vi "waveformprepare.vi"(7 "1762 Expose (us)":dbl, 8 "Microwave Expose Time (us)":dbl, 9 "Pump Expose Time (us)":dbl=256.0 format="%.2f") -> (3 "digital waveform out":digitalwaveform(waveform)={"t0"=timestamp(0 s since 1904-01-01), "dt"=0.0, "Y"={"transitions"=[], "data"=[]}, "error"={"status"=FALSE, "code"=37421928, "source"=""}})   [LabVIEW 2009]
uses:
  <vilib>/Waveform/DWDTOps.llb/DWDT Append Digital Samples.vi
  <vilib>/Waveform/DWDTOps.llb/DWDT Append Digital Signals.vi
  <vilib>/Waveform/DWDTOps.llb/Digital Pattern Generator (Single Value).vi
  <vilib>/Waveform/DWDTOps.llb/DWDT Invert Digital.vi
panel:
  out "Mixed Signal Graph":digitalwaveform(graph)
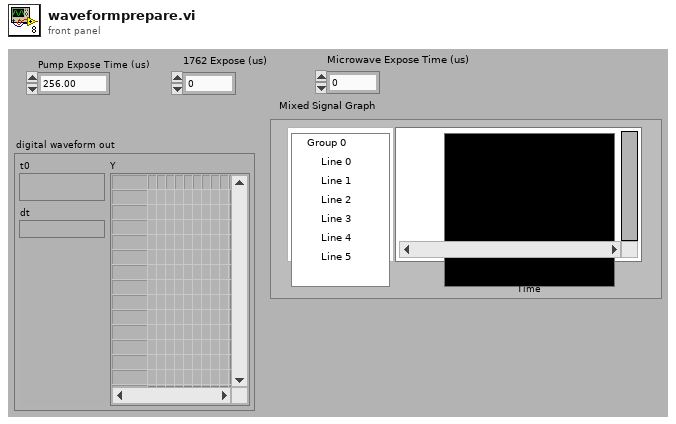
[diagram p1: front panel]
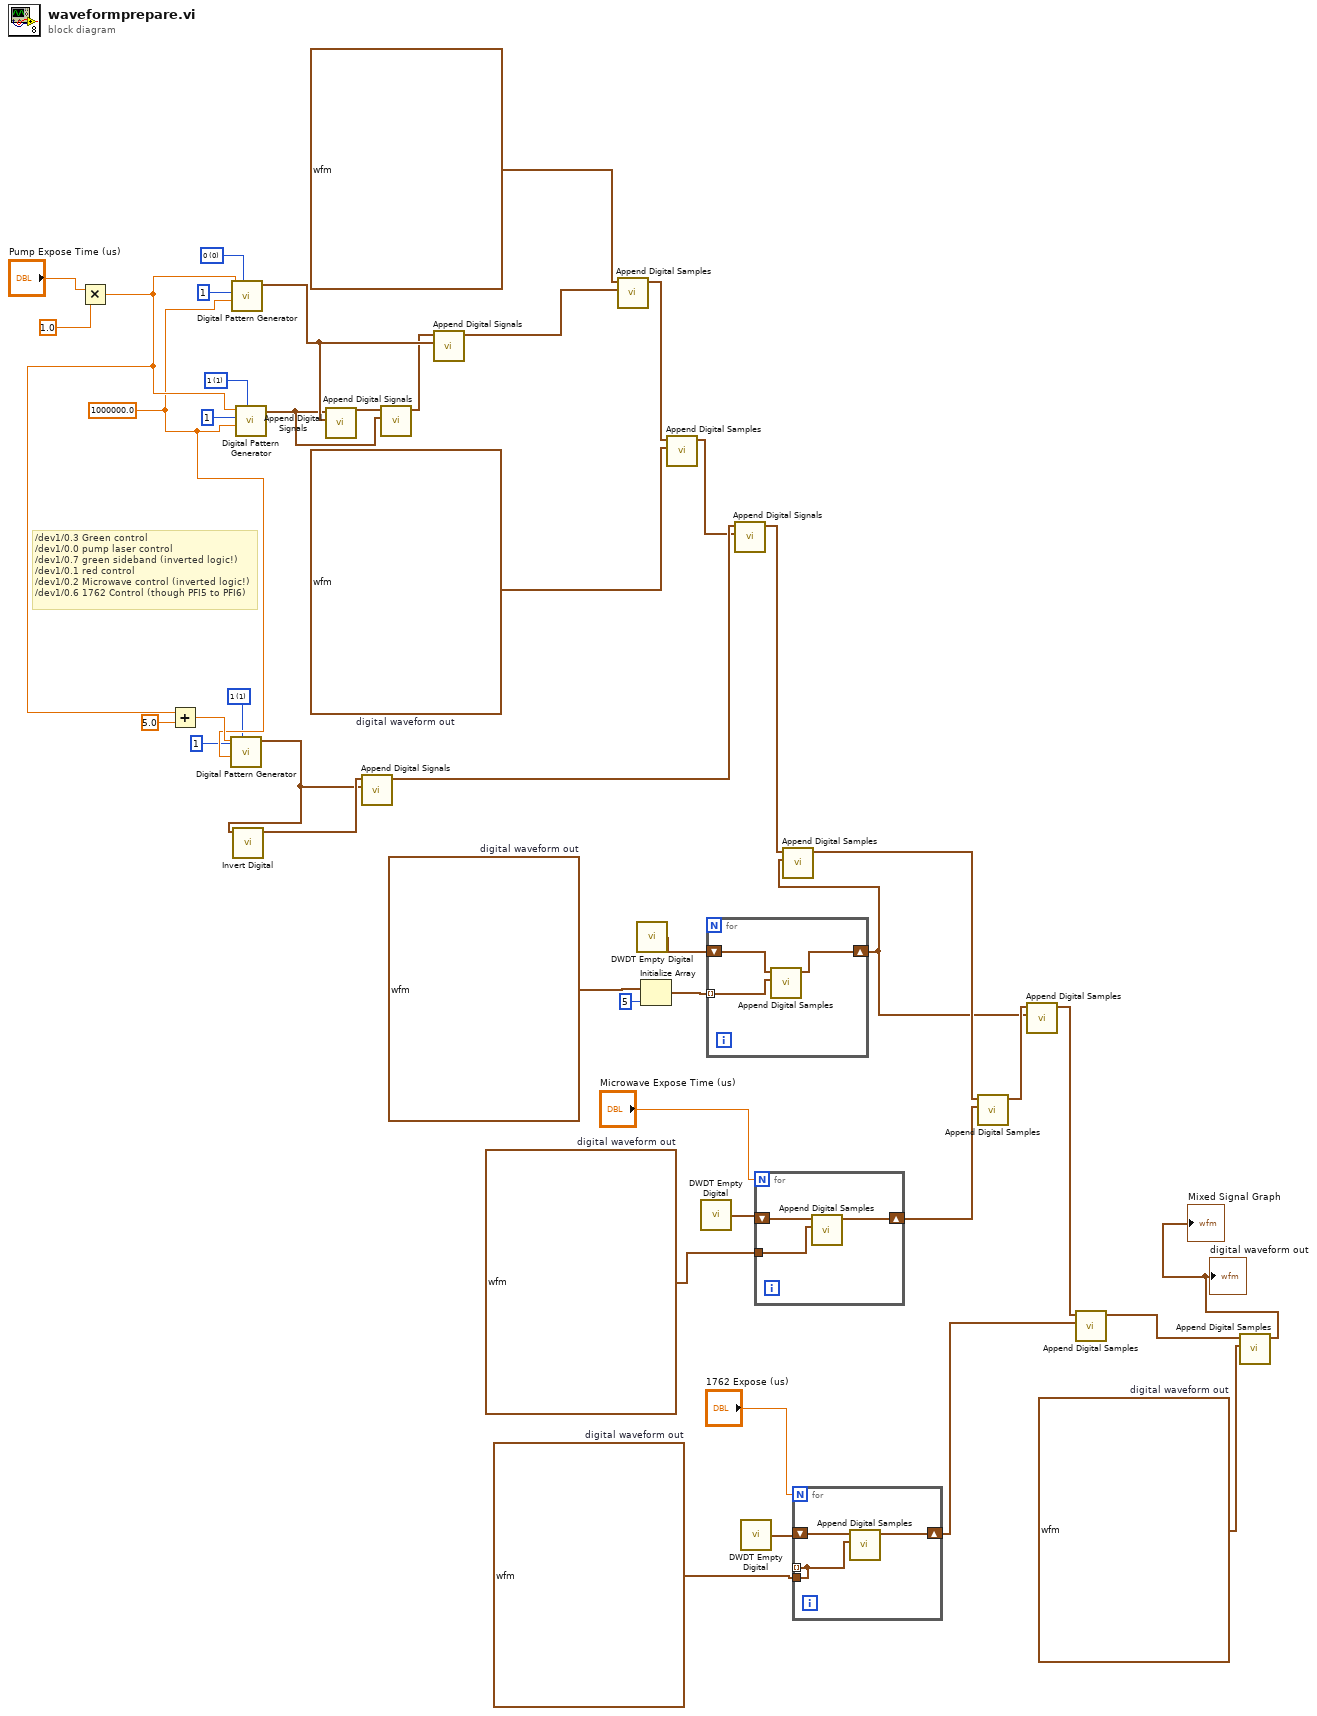
[diagram p0: block diagram]
diagram:
  w3 = digitalwaveform {"t0"=timestamp(0 s since 1904-01-01), "dt"=1e-06, "Y"={"transitions"=[], "data"=[[0, 1, 0, 1, 0, 0]]}, "error"={"status"=FALSE, "code"=37421928, "source"=""}}  # digital waveform out
  w11 = digitalwaveform {"t0"=timestamp(0 s since 1904-01-01), "dt"=1e-06, "Y"={"transitions"=[], "data"=[[1, 1, 0, 1, 0, 0]]}, "error"={"status"=FALSE, "code"=37421928, "source"=""}}  # digital waveform out
  w15 = digitalwaveform {"t0"=timestamp(0 s since 1904-01-01), "dt"=1e-06, "Y"={"transitions"=[], "data"=[[0, 0, 0, 1, 0, 0]]}, "error"={"status"=FALSE, "code"=37421928, "source"=""}}  # digital waveform out
  w19 = digitalwaveform {"t0"=timestamp(0 s since 1904-01-01), "dt"=1e-06, "Y"={"transitions"=[], "data"=[[0, 1, 0, 1, 0, 0]]}, "error"={"status"=FALSE, "code"=37421928, "source"=""}}  # digital waveform out
  w26 = u8 1 items=["0", "1", "Z", "L", "H", "X", "T", "V"] ("value")
  w39 = u8 1 items=["0", "1", "Z", "L", "H", "X", "T", "V"] ("value")
  w41 = u8 0 items=["0", "1", "Z", "L", "H", "X", "T", "V"] ("value")
  w27 = 1000000.0 ("sample rate")
  w42 = digitalwaveform {"t0"=timestamp(0 s since 1904-01-01), "dt"=1e-06, "Y"={"transitions"=[], "data"=[[1, 1, 1, 0], [1, 1, 0, 0], [1, 1, 0, 0], [1, 1, 0, 0], [1, 1, 0, 0], [1, 1, 0, 0], [1, 1, 0, 0], [1, 1, 0, 0], [1, 1, 0, 0], [1, 1, 0, 0], [0, 1, 0, 0]]}, "error"={"status"=FALSE, "code"=37421928, "source"=""}}  # digital waveform out
  # "/dev1/0.3 Green control\n/dev1/0.0 pump laser control\n/dev1/0.7 green sideband (inverted logic!)\n/dev1/0.1 red control\n/dev1/0.2 Microwave control (inverted logic!)\n/dev1/0.6 1762 Control (though PFI5 to PFI6)"
  n1 = Multiply(x="Pump Expose Time (us)", y=1.0) -> (x*y=w30:dbl)
  n2 = Add(x=w30, y=5.0) -> (x+y=w28:dbl)
  n3 = call-poly <vilib>:"Digital Pattern Generator.vi"("value"=w26, "sample rate"=w27, "number of signals"=u32 1, "number of samples"=w28) -> ("digital waveform"=w21:digitalwaveform)  [unwired: 6 in, 1 out]
  n4 = call-poly <vilib>:"Digital Pattern Generator.vi"("value"=w41, "sample rate"=w27, "number of signals"=u32 1, "number of samples"=w30) -> ("digital waveform"=w34:digitalwaveform)  [unwired: 6 in, 1 out]
  n5 = call-poly <vilib>:"Invert Digital.vi"("digital waveform"=w21) -> ("inverted waveform"=w22:digitalwaveform)  [unwired: 9 in, 1 out]
  n6 = call-poly <vilib>:"Digital Pattern Generator.vi"("value"=w39, "sample rate"=w27, "number of signals"=u32 1, "number of samples"=w30) -> ("digital waveform"=w32:digitalwaveform)  [unwired: 6 in, 1 out]
  n7 = call-poly <vilib>:"Append Digital Signals.vi"("digital waveform (low bits)"=w34, "digital waveform (high bits)"=w32) -> ("digital waveform out"=w33:digitalwaveform)  [unwired: 8 in, 1 out]
  n8 = call-poly <vilib>:"Append Digital Signals.vi"("digital waveform (low bits)"=w21, "digital waveform (high bits)"=w22) -> ("digital waveform out"=w24:digitalwaveform)  [unwired: 8 in, 1 out]
  n9 = call-poly <vilib>:"Append Digital Signals.vi"("digital waveform (low bits)"=w32, "digital waveform (high bits)"=w33) -> ("digital waveform out"=w31:digitalwaveform)  [unwired: 8 in, 1 out]
  n10 = call-poly <vilib>:"Append Digital Signals.vi"("digital waveform (low bits)"=w34, "digital waveform (high bits)"=w31) -> ("digital waveform out"=w38:digitalwaveform)  [unwired: 8 in, 1 out]
  n11 = call-poly <vilib>:"Append Digital Samples.vi"("digital waveform B"=w38, "digital waveform A"=digitalwaveform {"t0"=timestamp(0 s since 1904-01-01), "dt"=1e-06, "Y"={"transitions"=[], "data"=[[1, 0, 0, 1], [1, 0, 1, 0]]}, "error"={"status"=FALSE, "code"=37421928, "source"=""}} ("digital waveform out")) -> ("digital waveform out"=w35:digitalwaveform)  [unwired: 8 in, 1 out]
  n12 = call <vilib>:"DWDT Empty Digital.vi"() -> ("digital waveform out"=w16:digitalwaveform)  [unwired: 5 in]
  n13 = Initialize Array(w19, 5 ("dimension size")) -> (w17:digitalwaveform[])
  n14 = call-poly <vilib>:"Append Digital Samples.vi"("digital waveform B"=w42, "digital waveform A"=w35) -> ("digital waveform out"=w23:digitalwaveform)  [unwired: 8 in, 1 out]
  n15 = call <vilib>:"DWDT Empty Digital.vi"() -> ("digital waveform out"=w14:digitalwaveform)  [unwired: 5 in]
  n16 = for {
    tunnel: w17 -> [w47] mode=indexing
    shift-right: [w45] -> w5
    shift-left: w16 -> [w46]
    n17 = call-poly <vilib>:"Append Digital Samples.vi"("digital waveform B"=w47, "digital waveform A"=w46) -> ("digital waveform out"=w45:digitalwaveform)  [unwired: 8 in, 1 out]
  }
  n18 = call-poly <vilib>:"Append Digital Signals.vi"("digital waveform (low bits)"=w23, "digital waveform (high bits)"=w24) -> ("digital waveform out"=w20:digitalwaveform)  [unwired: 8 in, 1 out]
  n19 = call <vilib>:"DWDT Empty Digital.vi"() -> ("digital waveform out"=w10:digitalwaveform)  [unwired: 5 in]
  n20 = for {
    N: "Microwave Expose Time (us)" -> [_]
    tunnel: w15 -> [w50]
    shift-right: [w48] -> w13
    shift-left: w14 -> [w49]
    n21 = call-poly <vilib>:"Append Digital Samples.vi"("digital waveform B"=w50, "digital waveform A"=w49) -> ("digital waveform out"=w48:digitalwaveform)  [unwired: 8 in, 1 out]
  }
  n22 = call-poly <vilib>:"Append Digital Samples.vi"("digital waveform B"=w5, "digital waveform A"=w20) -> ("digital waveform out"=w12:digitalwaveform)  [unwired: 8 in, 1 out]
  n23 = for {
    N: "1762 Expose (us)" -> [_]
    tunnel: [w51] -> _ mode=indexing
    shift-right: [w52] -> w8
    shift-left: w10 -> [w53]
    tunnel: w11 -> [w51]
    n24 = call-poly <vilib>:"Append Digital Samples.vi"("digital waveform B"=w51, "digital waveform A"=w53) -> ("digital waveform out"=w52:digitalwaveform)  [unwired: 8 in, 1 out]
  }
  n25 = call-poly <vilib>:"Append Digital Samples.vi"("digital waveform B"=w13, "digital waveform A"=w12) -> ("digital waveform out"=w6:digitalwaveform)  [unwired: 8 in, 1 out]
  n26 = call-poly <vilib>:"Append Digital Samples.vi"("digital waveform B"=w5, "digital waveform A"=w6) -> ("digital waveform out"=w7:digitalwaveform)  [unwired: 8 in, 1 out]
  n27 = call-poly <vilib>:"Append Digital Samples.vi"("digital waveform B"=w8, "digital waveform A"=w7) -> ("digital waveform out"=w2:digitalwaveform)  [unwired: 8 in, 1 out]
  n28 = call-poly <vilib>:"Append Digital Samples.vi"("digital waveform B"=w3, "digital waveform A"=w2) -> ("digital waveform out"=→"digital waveform out" →"Mixed Signal Graph":digitalwaveform)  [unwired: 8 in, 1 out]
